vi "Event GUI QMH Template.vi"   [LabVIEW 2020, in "Volatus.lvlib"]
uses:
  Volatus.lvlib
  Module/Module.lvclass
  MessageQ/MessageQ.lvclass
types:
  T1 = enum32{"Invalid", "Standard", "Closed", "Hidden", "Minimized", "Maximized"}
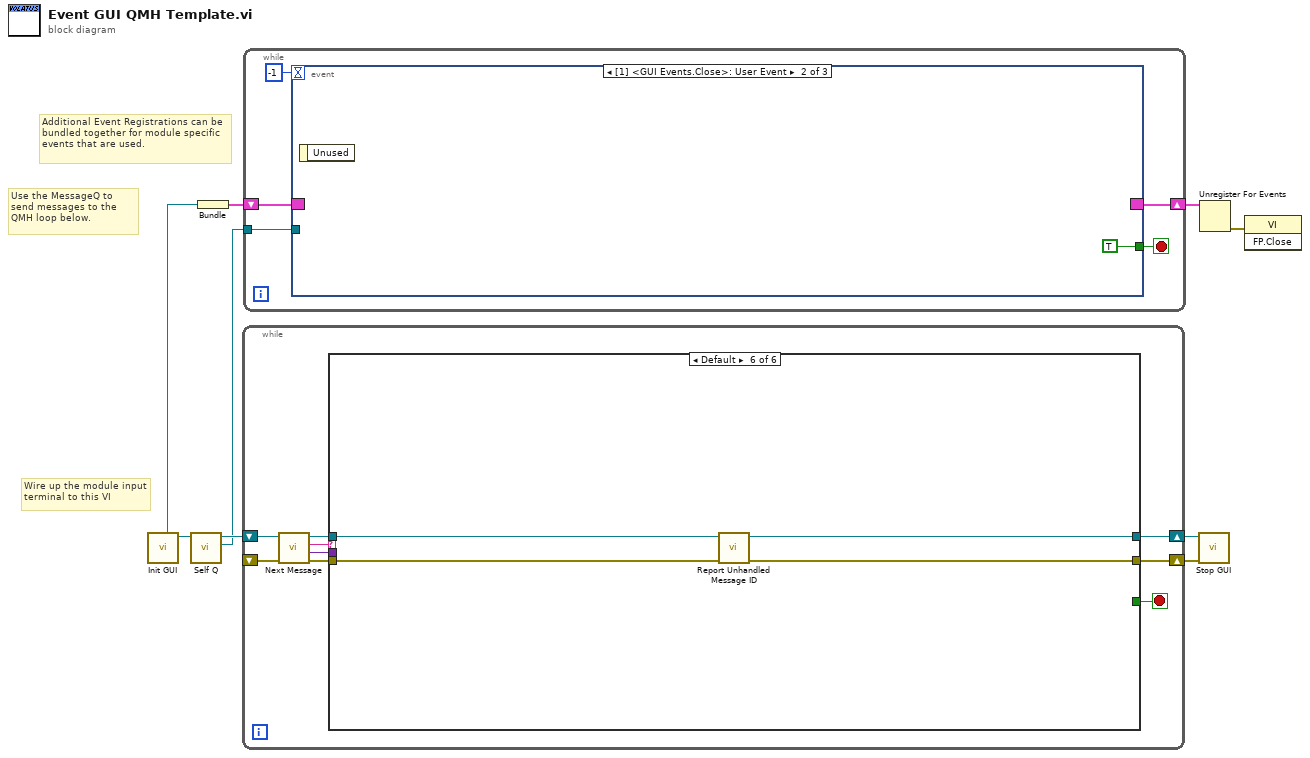
[diagram p0: block diagram]
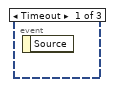
[diagram p2: hidden frame]
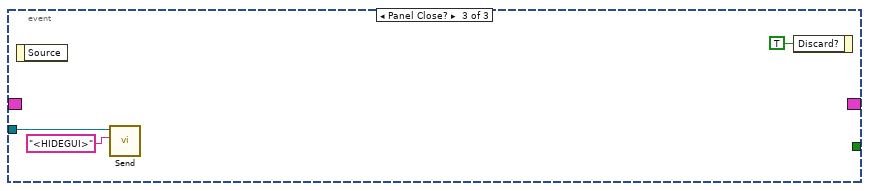
[diagram p3: hidden frame]
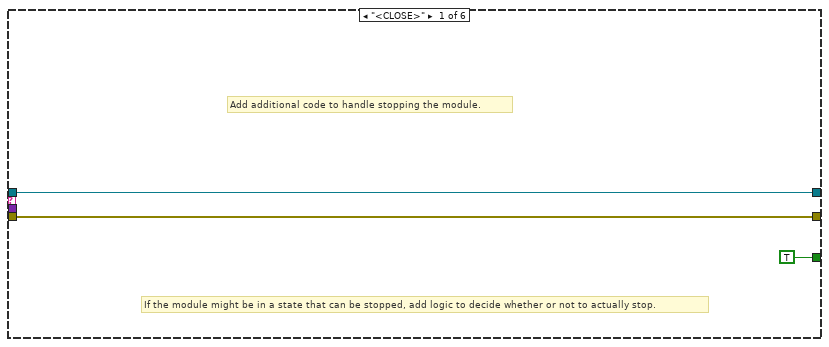
[diagram p4: hidden frame]
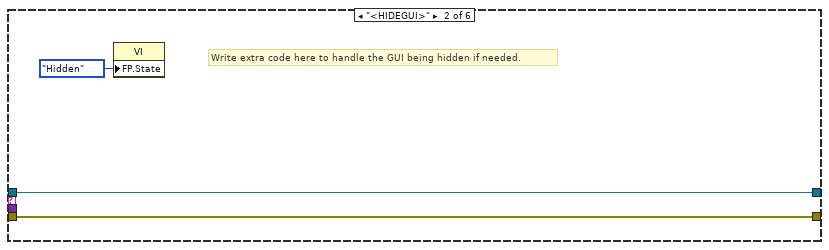
[diagram p5: hidden frame]
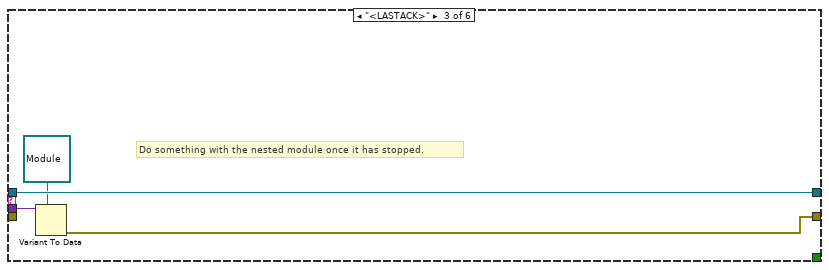
[diagram p6: hidden frame]
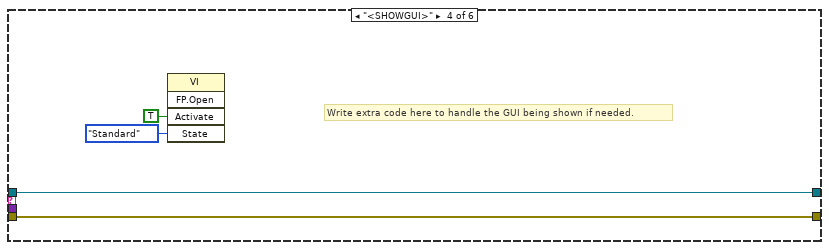
[diagram p7: hidden frame]
diagram:
  # "Additional Event Registrations can be bundled together for module specific events that are used."
  # "Use the MessageQ to send messages to the QMH loop below."
  # "Wire up the module input terminal to this VI"
  n1 = call "Init GUI.vi"() -> ("Module out"=w7:refnum<class "Module.lvclass">, "Event Reg"=w2:refnum<event-registration>)  [unwired: 10 in]
  n2 = call "Self Q.vi"("Module in"=w7) -> ("Self Q"=w8:refnum<class "MessageQ.lvclass">, "Module out"=w9:refnum<class "Module.lvclass">)  [unwired: 9 in]
  n3 = Bundle("Event Reg"=w2) -> (w6:cluster{"Event Reg":refnum<event-registration>})  [unwired: 1 in]
  n4 = while {
    shift-right: [w13] -> w4
    shift-left: w9 -> [w18]
    shift-right: [w12] -> w3
    shift-left: _ -> [w17]
    stop <- w11 stop-if-true
    n5 = call "Next Message.vi"("error in (no error)"=w17, "Module in"=w18) -> ("error out"=w16:errorcluster, "Data"=w10:variant, "ID"=w15:string, "Module out"=w14:refnum<class "Module.lvclass">)  [unwired: 6 in]
    n6 = case shown="Default" w15 {
      tunnel: w16 -> [w19 w23 _ w31 w33 w38]
      tunnel: w14 -> [w20 w24 w28 w32 w34 w36]
      tunnel: [w20 w24 w28 w32 w34 w35] -> w13
      tunnel: [w19 w23 w25 w31 w33 w37] -> w12
      tunnel: [TRUE _ _ _ _ _] -> w11
      tunnel: w10 -> [_ _ w27 _ _ _]
      frame "<CLOSE>" {
        # "If the module might be in a state that can be stopped, add logic to decide whether or not to actually stop."
        # "Add additional code to handle stopping the module."
      }
      frame "<HIDEGUI>" {
        # "Write extra code here to handle the GUI being hidden if needed."
        n7 = property class="VI"("FP.State"=T1."Hidden" ("Front Panel Window:State")) -> ()  [unwired: 2 in, 2 out]
      }
      frame "<LASTACK>" {
        # "Do something with the nested module once it has stopped."
        n8 = Variant To Data(type=refnum<class "Module.lvclass"> refnum ("Volatus:Module"), Variant=w27) -> (error out=w25:errorcluster)  [unwired: 1 in, 1 out]
      }
      frame "<SHOWGUI>" {
        # "Write extra code here to handle the GUI being shown if needed."
        n9 = invoke class="VI" method="FP.Open"("Activate"=TRUE ("Activate?"), "State"=T1."Standard") -> ()  [unwired: 3 in, 5 out]
      }
      frame "<TIMEOUT>" {
        # "No message for this module was received in time"
      }
      frame Default {
        n10 = call "Report Unhandled Message ID.vi"("error in (no error)"=w38, "Module in"=w36) -> ("error out"=w37:errorcluster, "Module out"=w35:refnum<class "Module.lvclass">)  [unwired: 8 in]
      }
    }
  }
  n11 = while {
    tunnel: w8 -> [w43]
    shift-right: [w41] -> w5
    shift-left: w6 -> [w42]
    stop <- w40 stop-if-true
    n12 = event shown="[1] <GUI Events.Close>: User Event" {
      selector: w42 -> [_ _ _]
      dyn-events: [_ _ _] -> w41
      timeout: -1 -> [_ _ _]
      tunnel: w43 -> [_ _ w46]
      tunnel: [_ TRUE _] -> w40
      event Timeout {
        n13 = event-data() -> ()  [unwired: 1 in, 1 out]
      }
      event User Event {
        n14 = event-data() -> ()  [unwired: 1 in, 1 out]
      }
      event Panel Close? {
        n15 = event-data() -> ()  [unwired: 1 in, 1 out]
        n16 = call "Send.vi"("ID"="<HIDEGUI>", "MessageQ in"=w46) -> ()  [unwired: 8 in, 2 out]
        n17 = event-data("Discard?"=TRUE) -> ()  [unwired: 1 in, 1 out]
      }
    }
  }
  n18 = call "Stop GUI.vi"("error in (no error)"=w3, "Module in"=w4) -> ()  [unwired: 8 in, 2 out]
  n19 = Unregister For Events(event registration refnum=w5) -> (error out=w1:errorcluster)  [unwired: 1 in]
  n20 = invoke class="VI" method="FP.Close"(error in=w1) -> ()  [unwired: 2 in, 3 out]
